vi "set_OSC.vi"   [LabVIEW 2012]
doc: "This vi reads the global variable and reads the contained data to the OSC. Make sure that you update the globals to the correct values before you use this vi!"
uses:
  global.vi
  libaries/Tektronix 7000 Series/Tektronix 7000 Series.lvlib
panel:
  # "SEE BLOCK DIAGRAM"
types:
  T1 = typedef "scale.ctl" = dbl
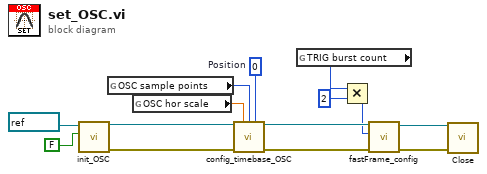
[diagram p0: block diagram]
diagram:
  w8 = 0  # Position
  n1 = call "init_OSC.vi"("reset (f)"=FALSE, "VISA resource name"=refnum<visa-resource-name> "OSC" ("OSC")) -> ("error out"=w14:errorcluster, "VISA resource name out"=w13:refnum<visa-resource-name>)  [unwired: 8 in]
  n2 = global read "global.vi" "OSC sample points"() -> (w10:i32)
  n3 = global read "global.vi" "OSC hor scale"() -> (w9:T1)
  n4 = call "config_timebase_OSC.vi"("VISA resource name"=w13, "hor scale"=w9, "resolution"=w10, "Position"=w8, "error in (no error)"=w14) -> ("VISA resource name out"=w7:refnum<visa-resource-name>, "error out"=w6:errorcluster)  [unwired: 9 in]
  n5 = global read "global.vi" "TRIG burst count"() -> (w3:i32)
  n6 = Multiply(x=w3, y=2) -> (x*y=w1:i32)
  n7 = call "fastFrame_config.vi"("error in (no error)"=w6, "fast frame count"=w1, "VISA resource name"=w7) -> ("error out"=w4:errorcluster, "VISA resource name out"=w5:refnum<visa-resource-name>)  [unwired: 7 in]
  n8 = call "Close.vi"("error in (no error)"=w4, "VISA resource name"=w5) -> ()  [unwired: 9 in, 1 out]
